vi "RichToFlatmicron_MessageReply.vi"(5 "OutputClusterType":T1, 11 "InputCluster":T3) -> (3 "OutputCluster":T1)   [LabVIEW 2019, in "Micron_client.lvlib"]
uses:
  Micron_client.lvlib
  micron_MessageReply.ctl
  micron_MessageReply_Status.ctl
  micron_MessageReply_Flat.ctl
  micron_MessageReply_Status_Flat.ctl
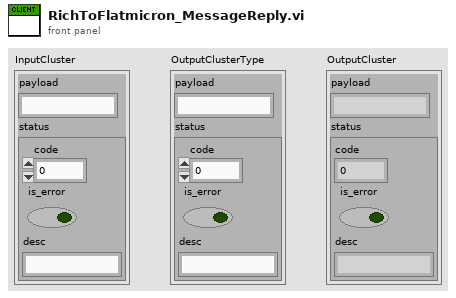
[diagram p1: front panel]
types:
  T1 = typedef "Micron_client.lvlib/micron_MessageReply_Flat.ctl" = cluster{"payload":string, "status":T2}
  T2 = typedef "Micron_client.lvlib/micron_MessageReply_Status_Flat.ctl" = cluster{"code":i32, "is_error":bool, "desc":string}
  T3 = typedef "Micron_client.lvlib/micron_MessageReply.ctl" = cluster{"payload":string, "status":T4}
  T4 = typedef "Micron_client.lvlib/micron_MessageReply_Status.ctl" = cluster{"code":i32, "is_error":bool, "desc":string}
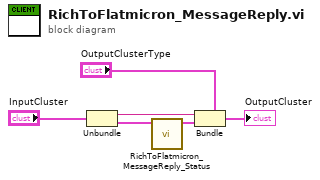
[diagram p0: block diagram]
diagram:
  n1 = Unbundle "Unbundle"("InputCluster") -> ("payload"=w3:string, "status"=w2:T4)
  n2 = call "RichToFlatmicron_MessageReply_Status.vi"("InputCluster"=w2) -> ("OutputCluster"=w1:T2)  [unwired: 10 in]
  n3 = Bundle "Bundle"(cluster="OutputClusterType", "payload"=w3, "status"=w1) -> (→"OutputCluster":T1)
